vi "moveMirror.vi"(6 "Delay between send and receive [ms]":i32=100, 8 "error in (no error)":errorcluster, 9 "position":i32, 10 "locationId":i32, 11 "Monochromator in":refnum<class "Monochromator.lvclass">) -> (0 "error out":errorcluster, 1 "ID":i32, 2 "results-JSON string":string, 3 "Monochromator out":refnum<class "Monochromator.lvclass">)   [LabVIEW 2023, in "horiba.lvlib" / "Monochromator.lvclass"]
doc: "Moves the specified mirror to a position.\n\nlocationId Integer. Identifies which mirror to move (zero-based).\n0 = Mirror 1 (Entrance)\n1 = Mirror 2 (Exit)\nposition Integer. Position to move to.\n0 = Axial\n1 = Lateral"
uses:
  Monochromator.lvclass
  f95066af-ee3f-403d-a38c-ce622af095b7.vi
  6615e9bd-2c56-4b02-b41e-62addde286d0.vi
  675900b5-fd1a-4005-b0fd-0124d8ccfa64.vi
  <vilib>/JDP Science/JSONtext/Variant to JSON Text.vi
  <vilib>/JDP Science/JSONtext/Set Item.vi
  <vilib>/JDP Science/JSONtext/LVClass Serializer/JSONtext LVClass Serializer.lvclass
  Monochromator.lvclass/Monochromator.ctl
  GenericDevice/GenericDevice.lvclass
  <vilib>/JDP Science/JSONtext/JSONtext.lvlib
panel:
  # "Connector Pane"
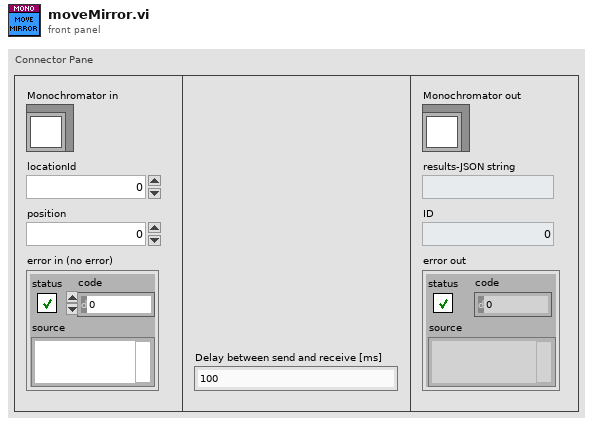
[diagram p1: front panel]
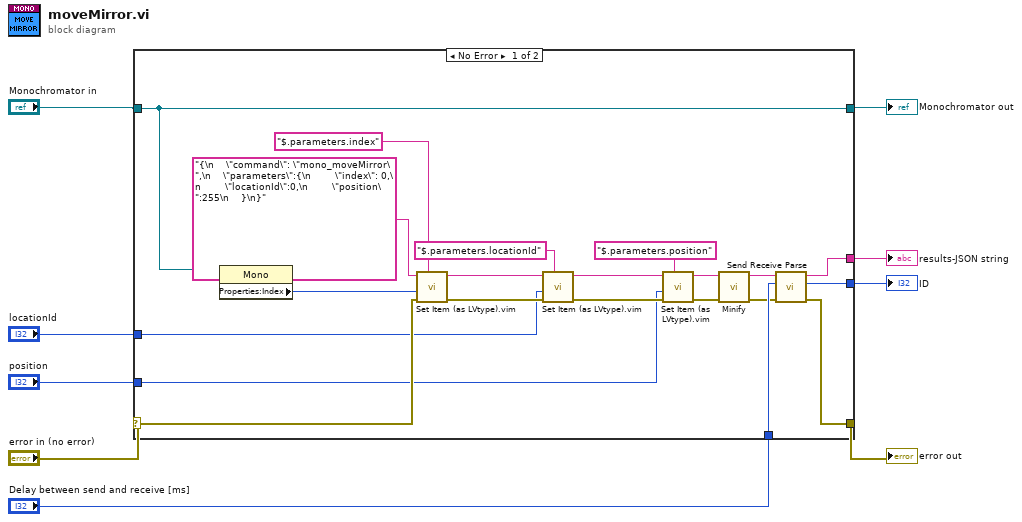
[diagram p0: block diagram]
diagram:
  n1 = case shown="No Error" "error in (no error)" {
    selector: "error in (no error)" -> [w26 w32]
    tunnel: [w23 w32] -> w6
    tunnel: [w28 w31] -> w8
    tunnel: "Monochromator in" -> [w28 w31]
    tunnel: [w25 _] -> w4
    tunnel: [w24 _] -> w5
    tunnel: "Delay between send and receive [ms]" -> [w15 _]
    tunnel: "locationId" -> [w14 _]
    tunnel: "position" -> [w13 _]
    frame No Error {
      n2 = property class="Mono"(reference=w28) -> ("Properties:Index"=w27:i32)  [unwired: 1 in, 2 out]
      n3 = call "Set Item (as LVtype).vim"("$Path or Item Name"="$.parameters.index", "error in (no error)"=w26, "Anything"=w27, "JSON"="{\n    \"command\": \"mono_moveMirror\",\n    \"parameters\":{\n        \"index\": 0,\n        \"locationId\":0,\n        \"position\":255\n    }\n}") -> ("error out"=w17:errorcluster, "<JSON>"=w19:string)  [unwired: 4 in, 1 out]
      n4 = call "Set Item (as LVtype).vim"("$Path or Item Name"="$.parameters.locationId", "error in (no error)"=w17, "Anything"=w14, "JSON"=w19) -> ("error out"=w16:errorcluster, "<JSON>"=w18:string)  [unwired: 4 in, 1 out]
      n5 = call "Set Item (as LVtype).vim"("$Path or Item Name"="$.parameters.position", "error in (no error)"=w16, "Anything"=w13, "JSON"=w18) -> ("error out"=w21:errorcluster, "<JSON>"=w11:string)  [unwired: 4 in, 1 out]
      n6 = call <vilib>:"Minify.vi"("error in (no error)"=w21, "JSON"=w11) -> ("error out"=w12:errorcluster, "<JSON>"=w10:string)  [unwired: 7 in, 1 out]
      n7 = call "Send Receive Parse.vi"("error in"=w12, "Delay between send and receive [ms]"=w15, "<JSON>"=w10) -> ("error out"=w23:errorcluster, "ID"=w24:i32, "results-JSON string"=w25:string)  [unwired: 6 in]
    }
    frame Error {
    }
  }
  "error out" <- w6
  "Monochromator out" <- w8
  "ID" <- w5
  "results-JSON string" <- w4
